vi "DLL Test.vi"() -> ()   [LabVIEW 2015]
panel:
  in  "dll Path":path
  in  "stop":bool
  in  "Run":bool
  in  "script path":string="C:\\Users\\tilin\\Desktop\\Vision_20160223\\Data\\Pattern"
  out "Data":string
  out "VAR":string
  out "length":i32
  out "string":string
  out "initialized array":u8[](array[numeric])
  out "DES":string
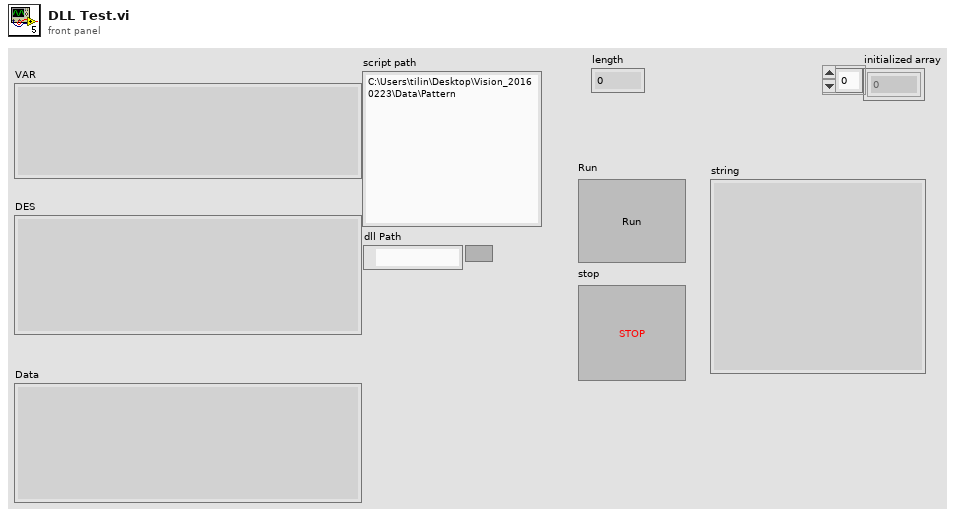
[diagram p1: front panel]
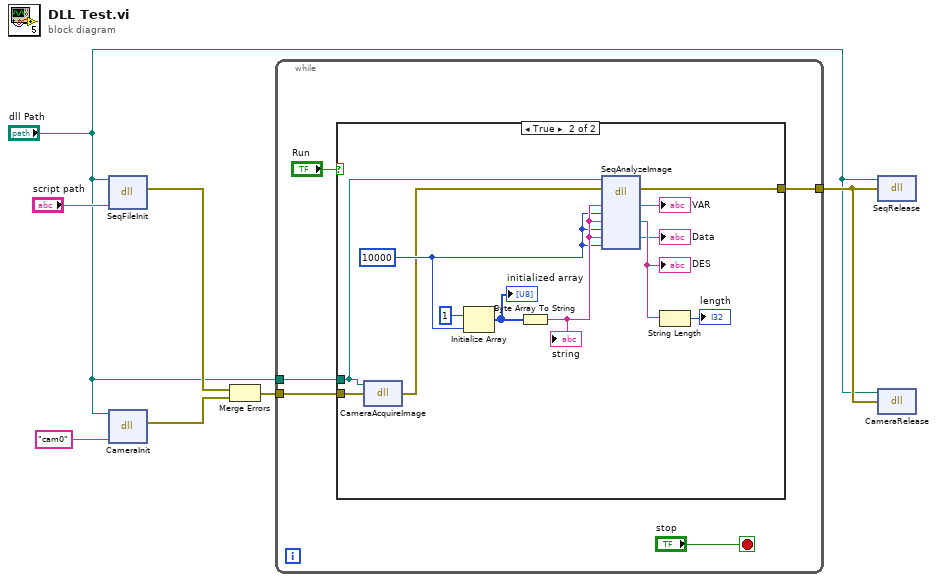
[diagram p0: block diagram]
diagram:
  n1 = dll-call lib="PTH2unc \n\\\\Mac\\Dropboxå²å¢ç§æè¡ä»½æéå¬å¸ç¨å¼é²åº¦[SourceCode] Source ControlVision_20160309DLLbuilds\nVisionSeq.dll" fn="SeqFileInit"(path in="dll Path", "scriptPath"="script path") -> (error out=w5:errorcluster)  [unwired: 4 in, 1 out]
  n2 = dll-call lib="PTH2unc \n\\\\Mac\\Dropboxå²å¢ç§æè¡ä»½æéå¬å¸ç¨å¼é²åº¦[SourceCode] Source ControlVision_20160309DLLbuilds\nVisionSeq.dll" fn="CameraInit"(path in="dll Path", "CameraName"="cam0") -> (error out=w4:errorcluster)  [unwired: 4 in, 1 out]
  n3 = Merge Errors(w5, w4) -> (w3:errorcluster)
  n4 = while {
    tunnel: w3 -> [w10]
    tunnel: [w9] -> w2
    tunnel: "dll Path" -> [w8]
    stop <- "stop" stop-if-true
    n5 = case shown="True" "Run" {
      tunnel: [w13 w25] -> w9
      tunnel: w10 -> [w13 w16]
      tunnel: w8 -> [_ w14]
      frame False {
      }
      frame True {
        w19 = 10000 ("Len")
        n6 = dll-call lib="PTH2unc \n\\\\Mac\\Dropboxå²å¢ç§æè¡ä»½æéå¬å¸ç¨å¼é²åº¦[SourceCode] Source ControlVision_20160309DLLbuilds\nVisionSeq.dll" fn="CameraAcquireImage"(path in=w14, error in=w16) -> (error out=w15:errorcluster)  [unwired: 2 in, 1 out]
        n7 = Initialize Array(1, w19) -> (w23:i32[])
        "initialized array" <- w23
        n8 = Byte Array To String(unsigned byte array=w23) -> (string=w20:string)
        "string" <- w20
        n9 = dll-call lib="PTH2unc \n\\\\Mac\\Dropboxå²å¢ç§æè¡ä»½æéå¬å¸ç¨å¼é²åº¦[SourceCode] Source ControlVision_20160309DLLbuilds\nVisionSeq.dll" fn="SeqAnalyzeImage"(path in=w14, error in=w15, "VarName"=w20, "VarName_Len"=w19, "description"=w20, "Description_Len"=w19, "Data"=w20, "Data_Len"=w19) -> (error out=w25:errorcluster, "VarName"=→"VAR":string, "description"=w21:string, "Data"=→"Data":string)  [unwired: 5 in, 1 out]
        "DES" <- w21
        n10 = String Length(string=w21) -> (length=→"length":i32)
      }
    }
  }
  n11 = dll-call lib="PTH2unc \n\\\\Mac\\Dropboxå²å¢ç§æè¡ä»½æéå¬å¸ç¨å¼é²åº¦[SourceCode] Source ControlVision_20160309DLLbuilds\nVisionSeq.dll" fn="SeqRelease"(path in="dll Path", error in=w2) -> ()  [unwired: 2 in, 2 out]
  n12 = dll-call lib="PTH2unc \n\\\\Mac\\Dropboxå²å¢ç§æè¡ä»½æéå¬å¸ç¨å¼é²åº¦[SourceCode] Source ControlVision_20160309DLLbuilds\nVisionSeq.dll" fn="CameraRelease"(path in="dll Path", error in=w2) -> ()  [unwired: 2 in, 2 out]
